vi "EndScript.vi"(8 "error in (no error)":errorcluster, 11 "VISA Refnum in":refnum<visa-resource-name>) -> (0 "error out":errorcluster, 2 "Tx for stopping code":string, 3 "VISA Refnum out":refnum<visa-resource-name>)   [LabVIEW 2016]
panel:
  out "Reply":string
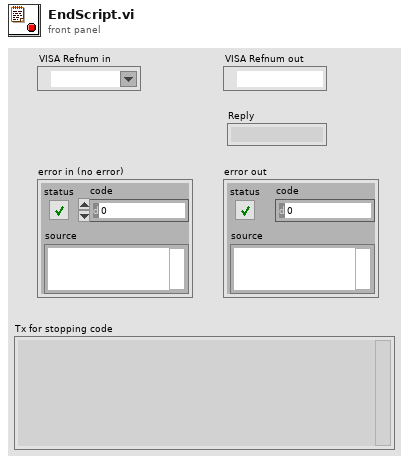
[diagram p1: front panel]
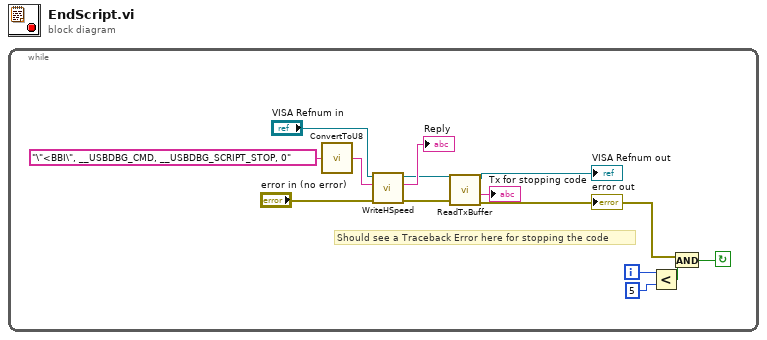
[diagram p0: block diagram]
diagram:
  n1 = while {
    i -> [w5]
    stop <- w1 continue-if-true
    # "Should see a Traceback Error here for stopping the code"
    n2 = call "ConvertToU8.vi"("struct"="\"<BBI\", __USBDBG_CMD, __USBDBG_SCRIPT_STOP, 0" ("write buffer")) -> ("Binary"=w10:string)
    n3 = call "WriteHSpeed.vi"("error in"="error in (no error)", "write buffer"=w10, "VISA Refnum in"="VISA Refnum in") -> ("error out"=w8:errorcluster, "read buffer"=→"Reply":string, "VISA Refnum out"=w7:refnum<visa-resource-name>)  [unwired: 6 in]
    n4 = call "ReadTxBuffer.vi"("error in"=w8, "VISA Refnum in"=w7) -> ("error out"=w2:errorcluster, "Tx Buffer"=→"Tx for stopping code":string, "VISA Refnum out"=→"VISA Refnum out":refnum<visa-resource-name>)  [unwired: 6 in, 1 out]
    "error out" <- w2
    n5 = Less?(x=w5, y=5) -> (x < y?=w3:bool)
    n6 = And(x=w2, y=w3) -> (x .and. y?=w1:bool)
  }
